vi "Prime BSI R3 Initialize.vi"(0 "Camera Handle":u32, 11 "Error":errorcluster) -> (15 "Error":errorcluster)   [LabVIEW 2016]
uses:
  Prime Controls/Prime ROI.ctl
panel:
  out "frames":u32=5341
  out "ADC Speed":i32=20000
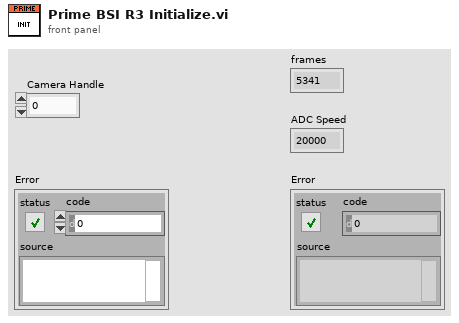
[diagram p1: front panel]
types:
  T1 = typedef "Prime ROI.ctl" = cluster{"X Start":u32, "X End":u32, "X Bin":u32, "Y Start":u32, "Y End":u32, "Y Bin":u32}
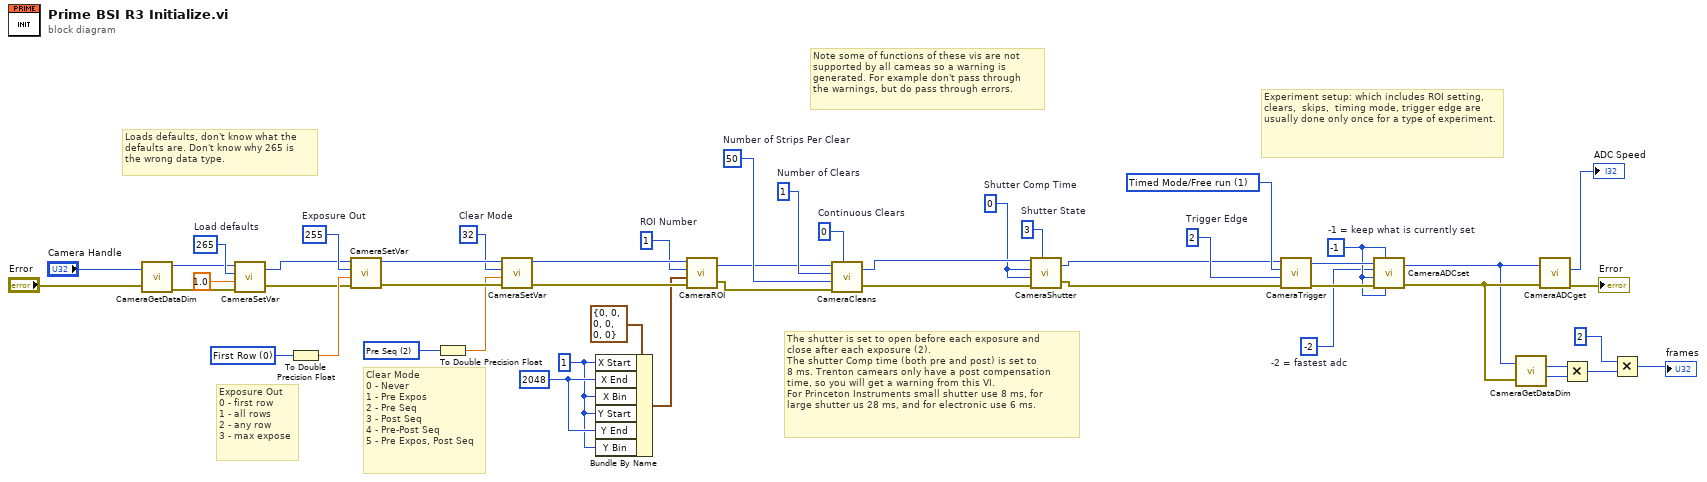
[diagram p0: block diagram]
diagram:
  w38 = u32 1 items=["N/A", "Timed Mode/Free run", "Trigger First (only PM)", "Strobed/Ext Sync"] ("Timing Mode")
  w9 = u32 3  # Shutter State
  w10 = u32 0  # Shutter Comp Time
  w14 = u32 1  # Number of Clears
  w15 = u32 50  # Number of Strips Per Clear
  w13 = u32 0  # Continuous Clears
  w18 = u32 2048 ("X End")
  w17 = u32 1 ("X Start")
  w27 = u32 2 items=["Never", "Pre Expos", "Pre Seq", "Post Seq", "Pre-Post Seq", "Pre Expos, Post Seq"] ("Clear Mode")
  w30 = u32 0 items=["First Row", "All Rows", "Any Row", "Max Exposure"] ("Exposure Out")
  w21 = u32 1  # ROI Number
  w26 = u32 32  # Clear Mode
  w28 = u32 255  # Exposure Out
  w39 = -2  # -2 = fastest adc
  w40 = -1  # -1 = keep what is currently set
  w43 = u32 2  # Trigger Edge
  w48 = u32 265  # Load defaults
  # "Note some of functions of these vis are not \nsupported by all cameas so a warning is \ngenerated. For example don't pass through \nthe warnings, but do pass through errors."
  # "The shutter is set to open before each exposure and\nclose after each exposure (2).\nThe shutter Comp time (both pre and post) is set to \n8 ms. Trenton camears only have a post compensation \ntime, so you will get a warning from this VI.\nFor Princeton Instruments small shutter use 8 ms, for \nlarge shutter us 28 ms, and for electronic use 6 ms."
  # "Clear Mode\n0 - Never\n1 - Pre Expos\n2 - Pre Seq\n3 - Post Seq\n4 - Pre-Post Seq\n5 - Pre Expos, Post Seq"
  # "Exposure Out\n0 - first row\n1 - all rows\n2 - any row\n3 - max expose"
  # "Experiment setup: which includes ROI setting, clears,  skips,  timing mode, trigger edge are usually done only once for a type of experiment."
  # "Loads defaults, don't know what the\ndefaults are. Don't know why 265 is\nthe wrong data type."
  n1 = call <userlib>:"CameraGetDataDim.vi"("Camera Handle"="Camera Handle", "error in"="Error") -> ("Camera Handle"=w45:u32, "error out"=w44:errorcluster)  [unwired: 2 out]
  n2 = call <userlib>:"CameraSetVar.vi"("error in"=w44, "Value"=1.0, "Parameter ID"=w48, "Camera Handle"=w45) -> ("error out"=w2:errorcluster, "CameraHandle"=w3:u32)
  n3 = To Double Precision Float(number=w30) -> (double precision float=w29:dbl)
  n4 = call <userlib>:"CameraSetVar.vi"("error in"=w2, "Value"=w29, "Parameter ID"=w28, "Camera Handle"=w3) -> ("error out"=w32:errorcluster, "CameraHandle"=w31:u32)
  n5 = To Double Precision Float(number=w27) -> (double precision float=w20:dbl)
  n6 = call <userlib>:"CameraSetVar.vi"("error in"=w32, "Value"=w20, "Parameter ID"=w26, "Camera Handle"=w31) -> ("error out"=w23:errorcluster, "CameraHandle"=w22:u32)
  n7 = Bundle By Name(cluster=T1 {"X Start"=0, "X End"=0, "X Bin"=0, "Y Start"=0, "Y End"=0, "Y Bin"=0} ("ROI Setup"), "X Start"=w17, "X End"=w18, "X Bin"=w17, "Y Start"=w17, "Y End"=w18, "Y Bin"=w17) -> (w16:T1)
  n8 = call <userlib>:"CameraROI.vi"("error in"=w23, "ROI Params"=w16, "ROI Index"=w21, "Camera Handle"=w22) -> ("error out"=w8:errorcluster, "Camera Handle"=w7:u32)
  n9 = call <userlib>:"CameraCleans.vi"("Camera Handle"=w7, "Number of Clears"=w14, "Number of Strips Per Clear"=w15, "error in"=w8, "Continuous Clears"=w13) -> ("Camera Handle"=w11:u32, "error out"=w12:errorcluster)
  n10 = call <userlib>:"CameraShutter.vi"("Camera Handle"=w11, "Shutter Comp Time: Pre Open"=w10, "Shutter Comp Time: Post Open"=w10, "error in"=w12, "Shutter State"=w9) -> ("Camera Handle"=w6:u32, "error out"=w5:errorcluster)
  n11 = call <userlib>:"CameraTrigger.vi"("error in"=w5, "Trigger Edge"=w43, "Timing Mode"=w38, "Camera Handle"=w6) -> ("error out"=w42:errorcluster, "Camera Handle"=w41:u32)
  n12 = call <userlib>:"CameraADCset.vi"("ADC offset"=w40, "Read Out port"=w40, "error in (no error)"=w42, "ADC Gain"=w40, "ADC Speed"=w39, "Camera Handle"=w41) -> ("error out"=w25:errorcluster, "Camera Handle"=w24:u32)
  n13 = call <userlib>:"CameraGetDataDim.vi"("Camera Handle"=w24, "error in"=w25) -> ("Xdim"=w4:u32, "Ydim"=w36:u32)  [unwired: 2 out]
  n14 = call <userlib>:"CameraADCget.vi"("Camera handle"=w24, "error in (no error)"=w25) -> ("ADC Speed"=→"ADC Speed":i32, "error out"=→"Error":errorcluster)  [unwired: 6 out]
  n15 = Multiply(x=w4, y=w36) -> (x*y=w34:u32)
  n16 = Multiply(x=u32 2, y=w34) -> (x*y=→"frames":u32)
